vi "sub vi - InitializeDDS.vi"(2 "timeout (ms)":u32=10000, 4 "End read on termination character?":bool=TRUE, 5 "data bits":u16=8 min=5 max=8 step=1, 6 "flow control":u16(ring) items=["None"=0, "XON/XOFF"=1, "RTS/CTS"=2, "DTR/DSR"=4], 7 "termination char\n(0xA = '\\n' = LF)":u8=10, 8 "stop bits":u16(ring)=10 items=["1.0"=10, "1.5"=15, "2.0"=20], 9 "parity":u16(ring) items=["None", "Odd", "Even", "Mark", "Space"], 10 "baud rate":u32=19200, 11 "VISA resource name":refnum<visa-resource-name>="COM22") -> (0 "error out":errorcluster, 3 "reference out":refnum<visa-resource-name>)   [LabVIEW 2010]
uses:
  <vilib>/Instr/_visa.llb/VISA Configure Serial Port (Instr).vi
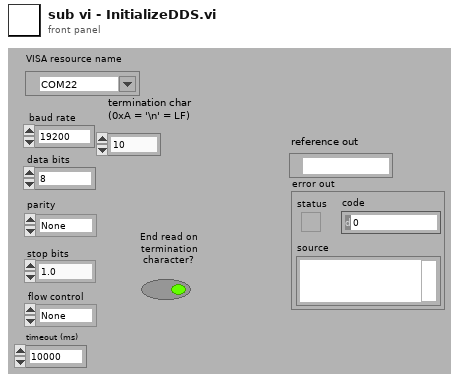
[diagram p1: front panel]
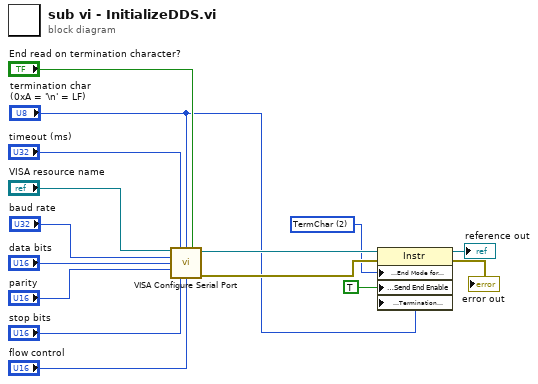
[diagram p0: block diagram]
diagram:
  w5 = u16 2 items=["None", "LastBit", "TermChar", "Break"] ("Serial Settings:Serial End Mode for Writes")
  n1 = call-poly "VISA Configure Serial Port"("VISA resource name"="VISA resource name", "timeout (10sec)"="timeout (ms)", "termination char\n(0xA = '\\n' = LF)"="termination char\n(0xA = '\\n' = LF)", "Enable Termination\nChar (T)"="End read on termination character?", "baud rate (9600)"="baud rate", "data bits (8)"="data bits", "parity (0:none)"="parity", "stop bits (10: 1 bit)"="stop bits", "flow control (0:none)"="flow control") -> ("VISA resource name out"=w6:refnum<visa-resource-name>, "error out"=w7:errorcluster)  [unwired: 1 in, 4 out]
  n2 = property class="Instr"(reference=w6, error in=w7, "Serial Settings:End Mode for Writes"=w5, "Message Based Settings:Send End Enable"=TRUE, "Message Based Settings:Termination Character"="termination char\n(0xA = '\\n' = LF)") -> (reference out=→"reference out":refnum<visa-resource-name>, error out=→"error out":errorcluster)
